vi "Read Range.vi"(8 "error in (no error)":errorcluster, 11 "Grove Ranging Sensor VL53L0X in":refnum<class "Grove Range Sensor VL53L0X .lvclass">) -> (0 "error out":errorcluster, 2 "Range":dbl, 3 "Grove Ranging Sensor VL53L0X out":refnum<class "Grove Range Sensor VL53L0X .lvclass">)   [LabVIEW 2020, in "CTI-Peripheral.lvlib" / "Grove Range Sensor VL53L0X .lvclass"]
uses:
  Grove Range Sensor VL53L0X .lvclass
  Grove Range Sensor VL53L0X .lvclass/Grove Range Sensor VL53L0X .ctl
  CTI/I2C Connection/I2C Connection.lvclass/I2C Connection.ctl
  CTI/Session/I2C Write Data.vi
  CTI/Session/I2C Read Data.vi
  CTI/I2C Connection/I2C Connection.lvclass
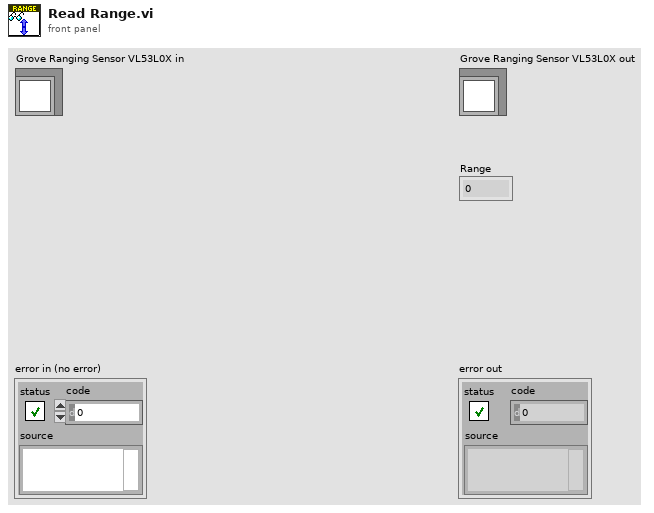
[diagram p1: front panel]
types:
  T1 = typedef "CTI-Peripheral.lvlib/Grove Range Sensor VL53L0X .lvclass/Range Mode.ctl" = enum16{"No Mode - Error", "Single", "Continuous", "High Speed", "High Accuracy", "Long Distance"}
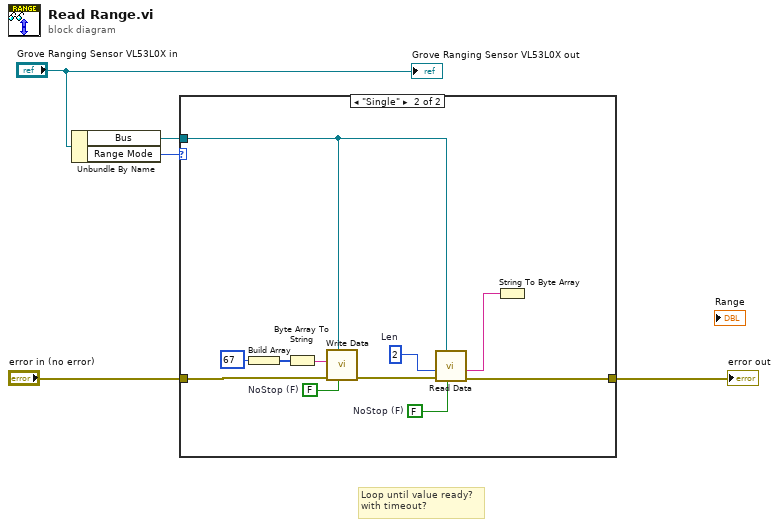
[diagram p0: block diagram]
diagram:
  # "Loop until value ready?\nwith timeout?"
  n1 = Unbundle By Name("Grove Ranging Sensor VL53L0X in") -> ("Bus"=w3:refnum<class "I2C Connection.lvclass">, "Range Mode"=w1:T1)
  n2 = case shown="\"Single\"" w1 {
    tunnel: "error in (no error)" -> [w6 w17]
    tunnel: w3 -> [_ w10]
    tunnel: [w6 w8] -> w2
    frame "No Mode - Error", Default {
    }
    frame "Single" {
      w11 = FALSE  # NoStop (F)
      w12 = u8 2  # Len
      w13 = FALSE  # NoStop (F)
      n3 = Build Array(u8 67 ("Register")) -> (w16:u8[])
      n4 = Byte Array To String(unsigned byte array=w16) -> (string=w14:string)
      n5 = call "Write Data.vi"("NoStop (F)"=w13, "I2C Connection"=w10, "error in (no error)"=w17, "Data"=w14) -> ("error out"=w9:errorcluster)  [unwired: 7 in]
      n6 = call "Read Data.vi"("NoStop (F)"=w11, "I2C Connection"=w10, "error in (no error)"=w9, "Len"=w12) -> ("error out"=w8:errorcluster, "Data"=w7:string)  [unwired: 6 in]
      n7 = String To Byte Array(string=w7) -> ()  [unwired: 1 out]
    }
  }
  "error out" <- w2
  "Grove Ranging Sensor VL53L0X out" <- "Grove Ranging Sensor VL53L0X in"
